vi "SlowControl.vi"(8 "Oscilloscope Ref":refnum<vi>, 9 "queue in":T2, 10 "notifier in":T1) -> ()   [LabVIEW 2022 SP3]
uses:
  TypeDefs/DataTypes/SystemStatus.ctl
  <vilib>/Waveform/WDTFileIO.llb/Export Waveforms To Spreadsheet File (1D).vi
  TypeDefs/QueueNotifier/DataQueue.ctl
  TypeDefs/QueueNotifier/Notifier.ctl
panel:
  in  "Open/Close Oscilloscope":bool
  in  "Delay Time (s)":dbl=1.0
  in  "stop 2":bool
  out "Error Message":string="No Error"
  out "Flow Integration":dbl(graph)
  out "LXe":dbl(slide) scale=0.0..2000.0
  out "Heater On/Off":bool
  in  "Allow Heater On?":bool
  in  "RTD1 Setpoint":dbl=165.0
  out "Flow, LJ channel 4":dbl(graph)
  out "Flow Rate":dbl=-0.039480482477756595
  out "Temperature Value 3":dbl=1411.5161689085326
  out "Temperature Value 4":dbl=-9725.85
  out "RTD1":dbl=-9725.85
  out "Temperature Value 2":dbl=-9725.85
  out "Temperature Value":dbl=-9725.85
  out "XY Graph 2":cluster{"Y":dbl[], "Y":dbl[]}[](graph) caption="Xenon Phase Diagram"
  out "XY Graph":cluster{"Y":dbl[], "Y":dbl[]}[](graph) caption="Xenon Phase Diagram"
  out "Bar":dbl=-0.2025818864027542
  out "Bar":dbl=-0.2025818864027542
  out "Torr":dbl=-0.2025818864027542
  out "Torr":dbl=-0.2025818864027542
  out "Pressure 2, LJ channel 2":dbl(graph)
  out "Pressure 1, LJ channel 8":dbl(graph)
  out "RTD 4, LJ channel 13 - Cell Top/SiPM":dbl(graph)
  out "RTD 3, LJ channel 12":dbl(graph)
  out "RTD 2, LJ channel 11":dbl(graph)
  out "RTD 1, LJ channel 10 - Cell Bottom":dbl(graph)
  out "RTD 0, LJ channel 1 - Coldfinger":dbl(graph)
  in  "File Path In":path=path "C:/Xe"
  in  "Error Button":bool
  in  "User's Error":errorcluster
  in  "Negative Channels":i32[](array[numeric])=[3, 5, 7, 9, 199, 199, 199, 199, 199, 199, 199]
  in  "Ranges":string[](array[string])=["LJ_rgBIP10V", "LJ_rgBIP10V", "LJ_rgBIP10V", "LJ_rgBIP10V", "LJ_rgBIP1V", "LJ_rgBIP1V", "LJ_rgBIP1V", "LJ_rgBIP1V", "LJ_rgBIP1V", "LJ_rgBIP1V", "LJ_rgBIP10V"]
  in  "Positive Channels":i32[](array[numeric])=[2, 4, 6, 8, 0, 1, 10, 11, 12, 13, 14]
  in  "Resolution":i32=10
  in  "SettlingFactor":i32=1
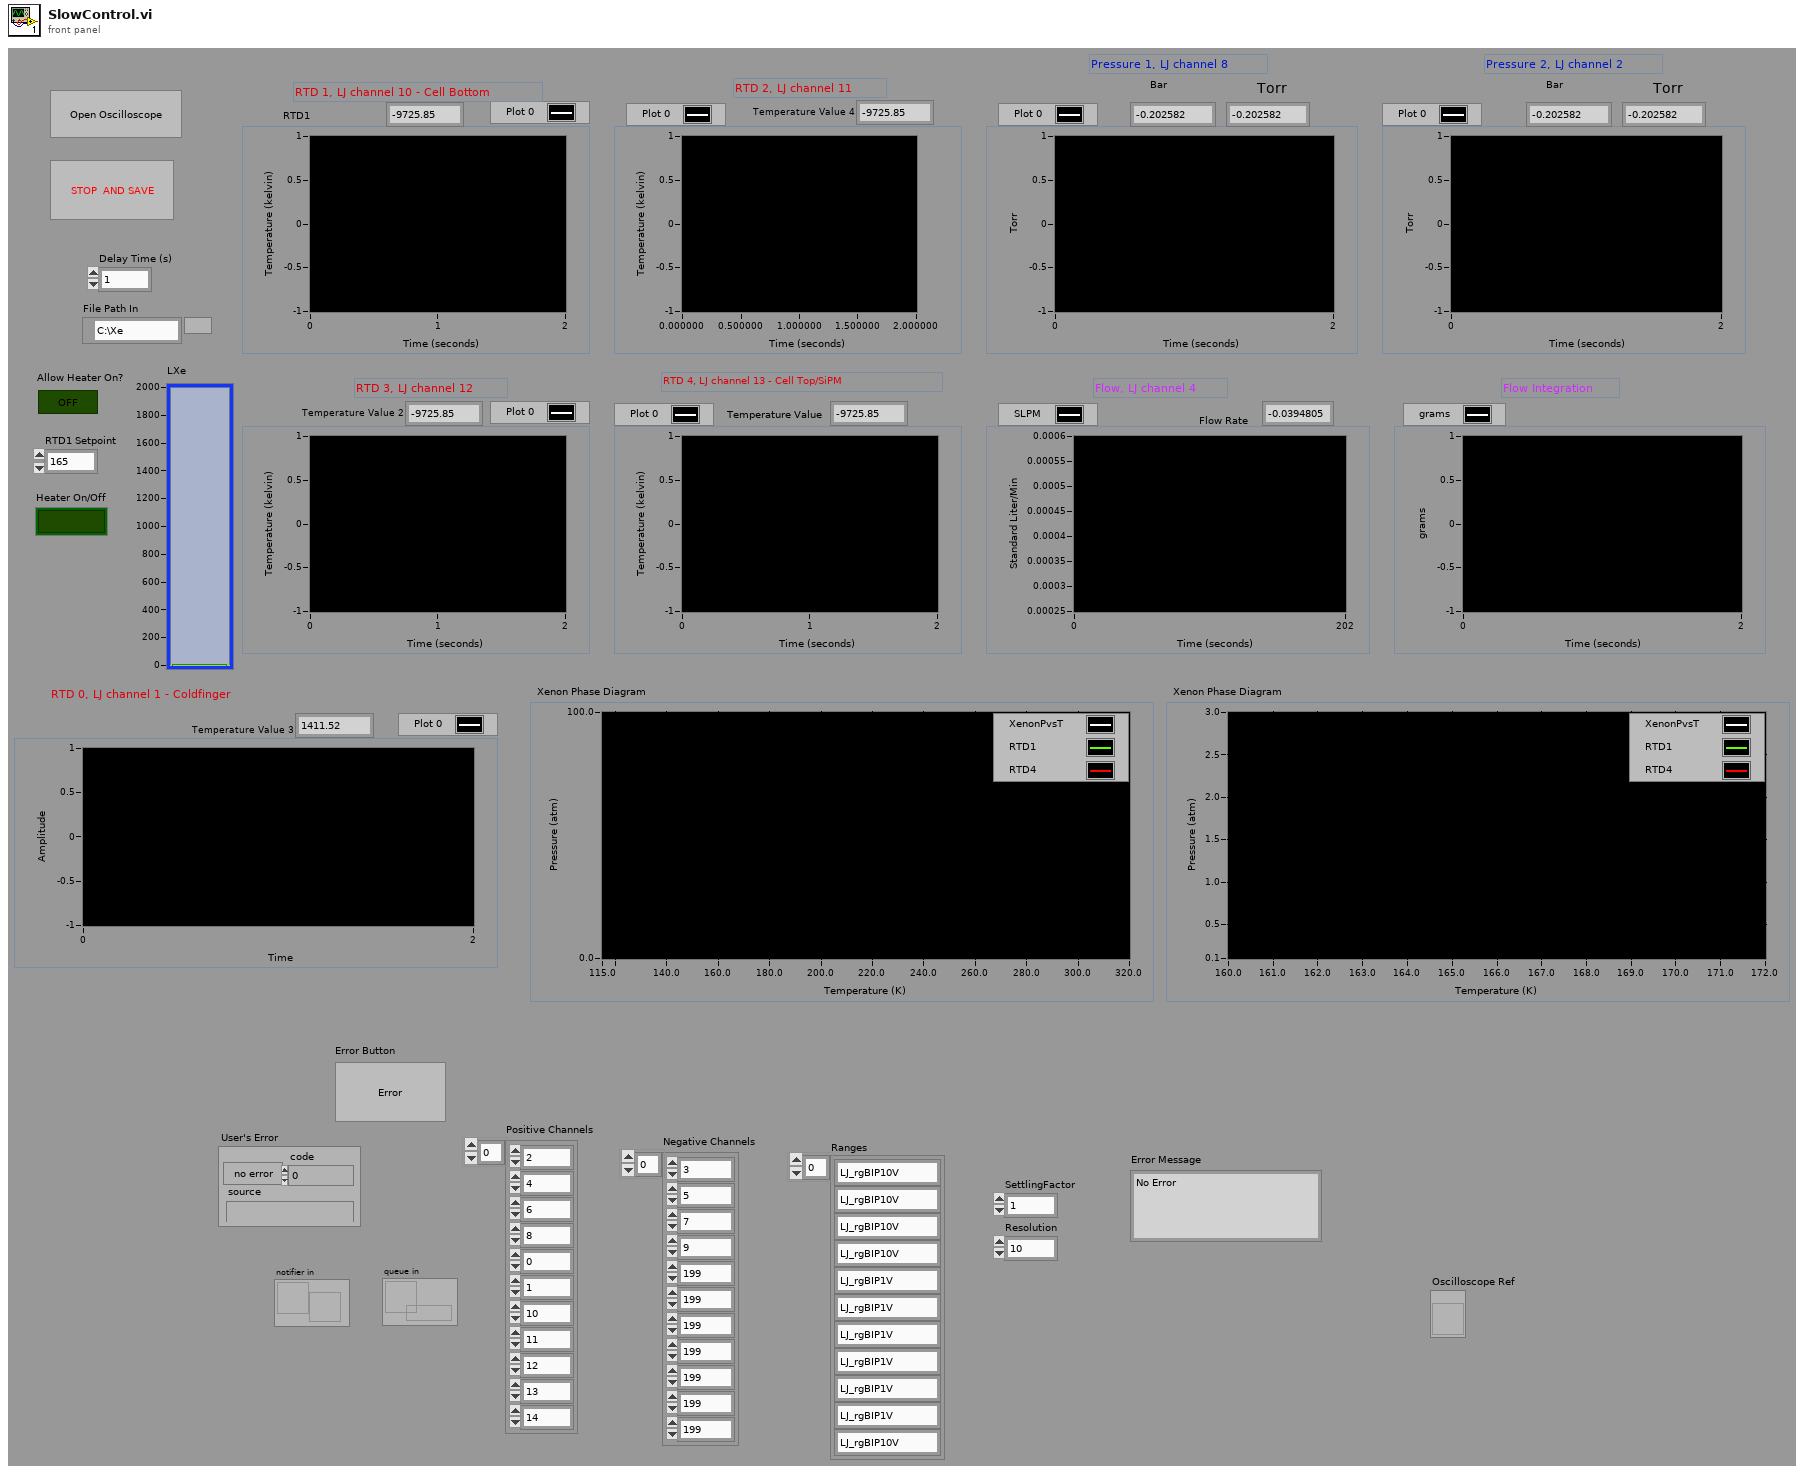
[diagram p1: front panel]
types:
  T1 = typedef "Notifier.ctl" = refnum<notifier>
  T2 = typedef "DataQueue.ctl" = refnum<queue>
  T3 = typedef "SystemStatus.ctl" = cluster{"Bias Voltage":dbl, "SiPM Temperature":dbl[], "Slow Control User":string, "LXe":dbl}
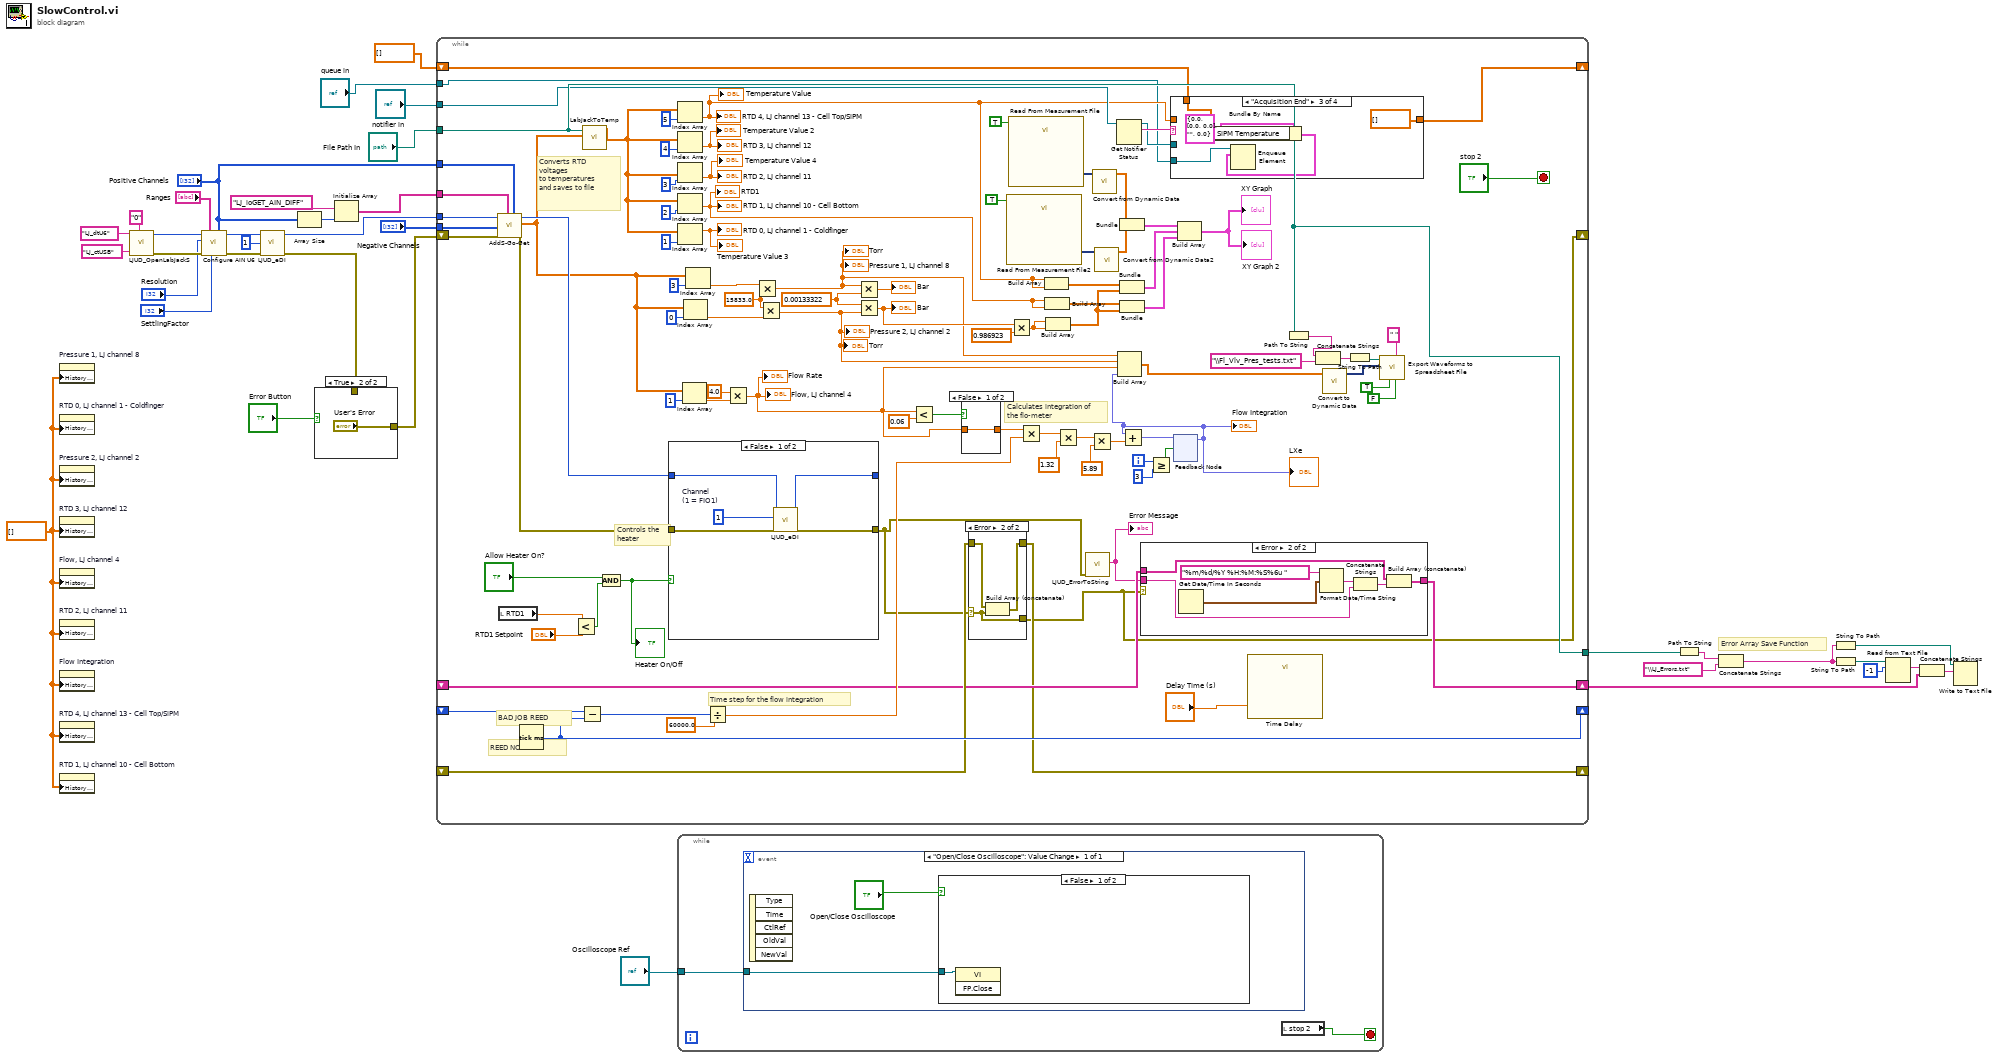
[diagram p0: block diagram]
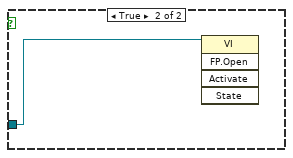
[diagram p2: hidden frame]
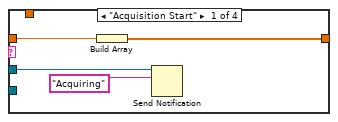
[diagram p3: hidden frame]
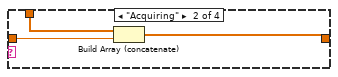
[diagram p4: hidden frame]
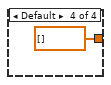
[diagram p5: hidden frame]
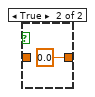
[diagram p8: hidden frame]
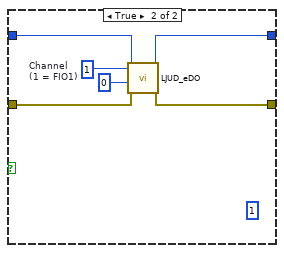
[diagram p9: hidden frame]
diagram:
  w5 = dbl[] [] ("History Data")
  # "Error Array Save Function"
  n1 = property on="Pressure 1, LJ channel 8" class="WFChart (strict)"("History Data"=w5) -> ()  [unwired: 2 in, 2 out]
  n2 = property on="RTD 0, LJ channel 1 - Coldfinger" class="WFChart (strict)"("History Data"=w5) -> ()  [unwired: 2 in, 2 out]
  n3 = property on="Pressure 2, LJ channel 2" class="WFChart (strict)"("History Data"=w5) -> ()  [unwired: 2 in, 2 out]
  n4 = property on="RTD 3, LJ channel 12" class="WFChart (strict)"("History Data"=w5) -> ()  [unwired: 2 in, 2 out]
  n5 = property on="Flow, LJ channel 4" class="WFChart (strict)"("History Data"=w5) -> ()  [unwired: 2 in, 2 out]
  n6 = property on="RTD 2, LJ channel 11" class="WFChart (strict)"("History Data"=w5) -> ()  [unwired: 2 in, 2 out]
  n7 = property on="Flow Integration" class="WFChart (strict)"("History Data"=w5) -> ()  [unwired: 2 in, 2 out]
  n8 = property on="RTD 4, LJ channel 13 - Cell Top/SiPM" class="WFChart (strict)"("History Data"=w5) -> ()  [unwired: 2 in, 2 out]
  n9 = property on="RTD 1, LJ channel 10 - Cell Bottom" class="WFChart (strict)"("History Data"=w5) -> ()  [unwired: 2 in, 2 out]
  n10 = call <vilib>:"LJUD_OpenLabJackS.vi"("Address"="0", "ConnectionType"="LJ_ctUSB", "DeviceType"="LJ_dtU6") -> ("error out"=w32:errorcluster, "Handle"=w33:i32)  [unwired: 6 in, 1 out]
  n11 = call <vilib>:"Configure AIN U6.vi"("Ranges"="Ranges", "SettlingFactor"="SettlingFactor", "Positive Channels"="Positive Channels", "error in"=w32, "Resolution"="Resolution", "Handle In"=w33) -> ("error out"=w28:errorcluster, "Handle Out"=w29:i32)  [unwired: 4 in]
  n12 = call <vilib>:"LJUD_eDI.vi"("error in"=w28, "Channel"=1, "Handle In"=w29) -> ("error out"=w17:errorcluster, "Handle Out"=w25:i32)  [unwired: 6 in, 1 out]
  n13 = Array Size(array="Positive Channels") -> (size(s)=w23:i32)
  n14 = case shown="True" "Error Button" {
    tunnel: [w37 "User's Error"] -> w18
    tunnel: w17 -> [w37 _]
    frame False {
    }
    frame True {
    }
  }
  n15 = Initialize Array("LJ_ioGET_AIN_DIFF" ("IOType"), w23) -> (w21:string[])
  n16 = while {
    tunnel: w25 -> [w134]
    tunnel: "Negative Channels" -> [w133]
    tunnel: w21 -> [w132]
    tunnel: "Positive Channels" -> [w131]
    tunnel: "File Path In" -> [w52]
    shift-right: [w87] -> _
    shift-left: _ -> [w88]
    shift-right: [w70] -> _
    shift-left: _ -> [w74]
    shift-right: [w48] -> _
    shift-left: w18 -> [w130]
    shift-right: [w72] -> w8
    shift-left: _ -> [w71]
    tunnel: [w52] -> w6
    tunnel: "notifier in" -> [w45]
    shift-right: [w42] -> _
    shift-left: dbl[] [] -> [w41]
    tunnel: "queue in" -> [w39]
    i -> [w51]
    stop <- "stop 2" stop-if-true
    w121 = 15833.0 ("y")
    w119 = 0.00133322 ("y")
    # "REED NO READ"
    # "BAD JOB REED"
    # "Time step for the flow integration"
    # "Converts RTD voltages \nto temperatures\nand saves to file"
    # "Calculates integration of\nthe flo-meter"
    # "Controls the \nheater"
    n17 = call <vilib>:"AddS-Go-Get.vi"("Channels"=w131, "IOTypes"=w132, "error in"=w130, "x1"=w133, "Handle In"=w134) -> ("error out"=w94:errorcluster, "Values Read"=w54:dbl[], "Handle Out"=w95:i32)  [unwired: 4 in]
    n18 = local read "RTD1"() -> (w93:dbl)
    n19 = Tick Count (ms)() -> (millisecond timer value=w87:u32)
    n20 = Less?(x=w93, y="RTD1 Setpoint") -> (x < y?=w91:bool)
    n21 = Subtract(x=w88, y=w87) -> (x-y=w85:u32)
    n22 = call "LabJackToTemp.vi"("LJ Data"=w54, "File Path"=w52) -> ("Temperatures"=w53:dbl[])  [unwired: 9 in]
    n23 = And(x="Allow Heater On?", y=w91) -> (x .and. y?=w89:bool)
    "Heater On/Off" <- w89
    n24 = case shown="False" w89 {
      tunnel: [w166 w169] -> w73
      tunnel: [w165 w168] -> _
      tunnel: w95 -> [w164 w171]
      tunnel: w94 -> [w163 w170]
      frame False {
        w167 = 1  # Channel (1 = FIO1)
        n25 = call <vilib>:"LJUD_eDI.vi"("error in"=w163, "Channel"=w167, "Handle In"=w164) -> ("error out"=w166:errorcluster, "Handle Out"=w165:i32)  [unwired: 6 in, 1 out]
      }
      frame True {
        (unwired) 1
        w172 = 1  # Channel (1 = FIO1)
        n26 = call <vilib>:"LJUD_eDO.vi"("error in"=w170, "State"=0, "Channel"=w172, "Handle In"=w171) -> ("error out"=w169:errorcluster, "Handle Out"=w168:i32)  [unwired: 6 in]
      }
    }
    n27 = Index Array(array=w53, index=5) -> (element=w43:dbl)
    "RTD 4, LJ channel 13 - Cell Top/SiPM" <- w43
    "Temperature Value" <- w43
    n28 = Index Array(array=w53, index=4) -> (element=→"RTD 3, LJ channel 12" →"Temperature Value 2":dbl)
    n29 = Index Array(array=w53, index=3) -> (element=→"RTD 2, LJ channel 11" →"Temperature Value 4":dbl)
    n30 = Index Array(array=w53, index=2) -> (element=w46:dbl)
    "RTD 1, LJ channel 10 - Cell Bottom" <- w46
    "RTD1" <- w46
    n31 = Index Array(array=w53, index=1) -> (element=→"RTD 0, LJ channel 1 - Coldfinger" →"Temperature Value 3":dbl)
    n32 = Index Array(array=w54, index=1) -> (element=w97:dbl)
    n33 = Index Array(array=w54, index=0) -> (element=w122:dbl)
    n34 = Index Array(array=w54, index=3) -> (element=w120:dbl)
    n35 = Divide(x=w85, y=60000.0) -> (x/y=w79:dbl)
    n36 = Multiply(x=4.0, y=w97) -> (x*y=w60:dbl)
    "Flow Rate" <- w60
    "Flow, LJ channel 4" <- w60
    n37 = Multiply(x=w120, y=w121) -> (x*y=w61:dbl)
    "Pressure 1, LJ channel 8" <- w61
    "Torr" <- w61
    n38 = Multiply(x=w121, y=w122) -> (x*y=w62:dbl)
    "Pressure 2, LJ channel 2" <- w62
    "Torr" <- w62
    n39 = Multiply(x=w61, y=w119) -> (x*y=→"Bar":dbl)
    n40 = Multiply(x=w119, y=w62) -> (x*y=w105:dbl)
    "Bar" <- w105
    n41 = Less?(x=w60, y=0.06) -> (x < y?=w83:bool)
    n42 = case shown="False" w83 {
      tunnel: w60 -> [w161 _]
      tunnel: [w161 0.0] -> w80
      frame False {
      }
      frame True {
      }
    }
    n43 = case shown="Error" w73 {
      selector: w73 -> [w157 w158]
      tunnel: [w157 w158] -> w48
      tunnel: [w156 w160] -> w70
      tunnel: w74 -> [w156 w159]
      frame No Error {
      }
      frame Error {
        n44 = Build Array (concatenate)(w159, w158) -> (w160:errorcluster[])
      }
    }
    n45 = call "Read From Measurement File2"("Reset"=TRUE) -> ("Signals"=w115:dynamicdata)  [unwired: 5 in, 5 out]
    n46 = call "Read From Measurement File"("Reset"=TRUE) -> ("Signals"=w114:dynamicdata)  [unwired: 5 in, 5 out]
    n47 = Multiply(x=w105, y=0.986923) -> (x*y=w106:dbl)
    n48 = Multiply(x=w80, y=w79) -> (x*y=w78:dbl)
    n49 = Build Array(w43, w43) -> (w103:dbl[])
    n50 = Build Array(w46, w46) -> (w102:dbl[])
    n51 = Build Array(w106, w106) -> (w104:dbl[])
    n52 = Multiply(x=w78, y=1.32) -> (x*y=w77:dbl)
    n53 = call <vilib>:"LJUD_ErrorToString.vi"("error in"=w73) -> ("String"=w69:string)  [unwired: 10 in]
    "Error Message" <- w69
    n54 = Multiply(x=w77, y=5.89) -> (x*y=w76:dbl)
    n55 = call "Convert from Dynamic Data"("Dynamic Data Type"=w114) -> ("Array"=w113:dbl[])  [unwired: 3 in]
    n56 = call "Convert from Dynamic Data2"("Dynamic Data Type"=w115) -> ("Array"=w112:dbl[])  [unwired: 3 in]
    n57 = Get Notifier Status(notifier=w45) -> (notifier out=w40:T1, current notification=w44:string)  [unwired: 1 in, 3 out]
    n58 = Bundle("Array"=w113, "Array"=w112) -> (w110:cluster{"Array":dbl[], "Array":dbl[]})  [unwired: 1 in]
    n59 = Bundle(w103, w104) -> (w109:cluster{dbl[], dbl[]})  [unwired: 1 in]
    n60 = Bundle(w102, w104) -> (w108:cluster{dbl[], dbl[]})  [unwired: 1 in]
    n61 = case shown="Error" w48 {
      tunnel: [w148 w154] -> w72
      tunnel: w71 -> [w148 w155]
      tunnel: w69 -> [_ w151]
      frame No Error {
      }
      frame Error {
        n62 = Get Date/Time In Seconds() -> (seconds since 1Jan1904=w153:timestamp)
        n63 = Format Date/Time String(time format string (%c)="%m/%d/%Y %H:%M:%S%6u ", seconds (now)=w153) -> (date/time string=w150:string)  [unwired: 1 in]
        n64 = Concatenate Strings(w150, w151) -> (w149:string)
        n65 = Build Array (concatenate)(w155, w149) -> (w154:string[])
      }
    }
    n66 = Greater Or Equal?(x=w51, y=3) -> (x >= y?=w49:bool)
    n67 = case shown="\"Acquisition End\"" w44 {
      tunnel: w43 -> [w138 w141 _ _]
      tunnel: [w137 w139 dbl[] [] dbl[] []] -> w42
      tunnel: w41 -> [_ w140 w143 _]
      tunnel: w40 -> [w136 _ _ _]
      tunnel: w39 -> [_ _ w145 _]
      frame "Acquisition Start" {
        n68 = Build Array(w138) -> (w137:dbl[])
        n69 = Send Notification(notification="Acquiring", notifier=w136) -> ()  [unwired: 1 in, 2 out]
      }
      frame "Acquiring" {
        n70 = Build Array (concatenate)(w140, w141) -> (w139:dbl[])
      }
      frame "Acquisition End" {
        n71 = Bundle By Name(cluster=T3 {"Bias Voltage"=0.0, "SiPM Temperature"=[0.0, 0.0], "Slow Control User"="", "LXe"=0.0} ("System Status"), "SiPM Temperature"=w143) -> (w142:T3)
        n72 = Enqueue Element(queue=w145, element=w142) -> ()  [unwired: 2 in, 3 out]
      }
      frame Default {
      }
    }
    n73 = feedback #1() -> (w59:fxp<+/-,32,16>)  [unwired: 1 in]
    "LXe" <- w59
    "Flow Integration" <- w59
    n74 = Build Array(w61, w62, w60, w59) -> (w58:dbl[])
    n75 = Add(x=w59, y=w76) -> (x+y=w75:fxp<+/-,32,16>)
    n76 = feedback-in #1(w75, w49) -> ()
    n77 = Build Array(w110, w109, w108) -> (→"XY Graph" →"XY Graph 2":cluster{"Array":dbl[], "Array":dbl[]}[])
    n78 = call "Time Delay"("Delay Time (s)"="Delay Time (s)") -> ()  [unwired: 10 in, 1 out]
    n79 = Path To String(path=w52) -> (string=w57:string)
    n80 = Concatenate Strings(w57, "\\Fl_Vlv_Pres_tests.txt") -> (w65:string)
    n81 = call "Convert to Dynamic Data"("Array"=w58) -> ("Dynamic Data Type"=w67:dynamicdata)  [unwired: 3 in]
    n82 = String To Path(string=w65) -> (path=w64:path)
    n83 = call-poly <vilib>:"Export Waveforms to Spreadsheet File.vi"("header? (write header:T)"=FALSE, "delimiter (Tab)"=" ", "append to file? (new file:F)"=TRUE, "waveforms"=w67, "file path (dialog if empty)"=w64) -> ()  [unwired: 5 in, 2 out]
  }
  n84 = while {
    tunnel: "Oscilloscope Ref" -> [w175]
    stop <- w174 stop-if-true
    n85 = event shown="[0] \"Open/Close Oscilloscope\": Value Change" {
      selector: _ -> [_]
      dyn-events: _ -> [_]
      timeout: _ -> [_]
      tunnel: w175 -> [w176]
      event "Open/Close Oscilloscope": Value Change {
        n86 = event-data() -> ()  [unwired: 1 in, 5 out]
        n87 = case shown="False" "Open/Close Oscilloscope" {
          tunnel: w176 -> [w178 w179]
          frame False {
            n88 = invoke class="VI" method="FP.Close"(reference=w178) -> ()  [unwired: 2 in, 3 out]
          }
          frame True {
            n89 = invoke class="VI" method="FP.Open"(reference=w179) -> ()  [unwired: 4 in, 5 out]
          }
        }
      }
    }
    n90 = local read "stop 2"() -> (w174:bool)
  }
  n91 = Path To String(path=w6) -> (string=w7:string)
  n92 = Concatenate Strings(w7, "\\LJ_Errors.txt") -> (w9:string)
  n93 = String To Path(string=w9) -> (path=w14:path)
  n94 = String To Path(string=w9) -> (path=w13:path)
  n95 = Read from Text File(file (use dialog)=w13, count=-1) -> (text=w11:string)  [unwired: 2 in, 3 out]
  n96 = Concatenate Strings(w11, w8) -> (w10:string)
  n97 = Write to Text File(file (use dialog)=w14, text=w10) -> ()  [unwired: 2 in, 3 out]
